vi "avg8.vi"(10 "Input":i16) -> (2 "Output":i16)   [LabVIEW 2018, in "kevLib2010.lvlib"]
uses:
  kevLib2010.lvlib
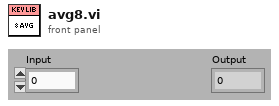
[diagram p1: front panel]
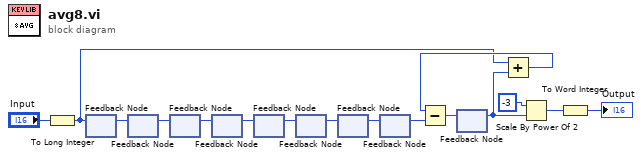
[diagram p0: block diagram]
diagram:
  n1 = To Long Integer(number="Input") -> (32bit integer=w3:i32)
  n2 = feedback-in #1(w3) -> ()
  n3 = feedback #1() -> (w16:i32)  [unwired: 1 in]
  n4 = feedback-in #2(w16) -> ()
  n5 = feedback #2() -> (w15:i32)  [unwired: 1 in]
  n6 = feedback-in #3(w15) -> ()
  n7 = feedback #3() -> (w14:i32)  [unwired: 1 in]
  n8 = feedback-in #4(w14) -> ()
  n9 = feedback #4() -> (w13:i32)  [unwired: 1 in]
  n10 = feedback-in #5(w13) -> ()
  n11 = feedback #5() -> (w12:i32)  [unwired: 1 in]
  n12 = feedback-in #6(w12) -> ()
  n13 = feedback #6() -> (w11:i32)  [unwired: 1 in]
  n14 = feedback-in #7(w11) -> ()
  n15 = feedback #7() -> (w6:i32)  [unwired: 1 in]
  n16 = feedback-in #8(w6) -> ()
  n17 = feedback #8() -> (w5:i32)  [unwired: 1 in]
  n18 = feedback #9() -> (w8:i32)  [unwired: 1 in]
  n19 = Add(x=w3, y=w8) -> (x+y=w10:i32)
  n20 = Subtract(x=w10, y=w5) -> (x-y=w9:i32)
  n21 = feedback-in #9(w9) -> ()
  n22 = Scale By Power Of 2(n=-3, x=w8) -> (x*2^n=w2:i32)
  n23 = To Word Integer(number=w2) -> (16bit integer=→"Output":i16)
